vi "Big Temp Read and Test.vi"(7 "Initialize":bool, 8 "Error In":errorcluster, 9 "Cluster":T1, 10 "Cycle Time (S)":dbl, 11 "VISA resource name":refnum<visa-resource-name>) -> (0 "Error Out":errorcluster, 1 "Readout":dbl, 2 "Blinking":bool, 3 "VISA resource name":refnum<visa-resource-name>)   [LabVIEW 2021]
uses:
  <vilib>/Analysis/3filter.llb/Filter Passband Type.ctl
  <vilib>/Analysis/NI_AALBase.lvlib
  <vilib>/ptbypt/NI_PtbyPt.lvlib
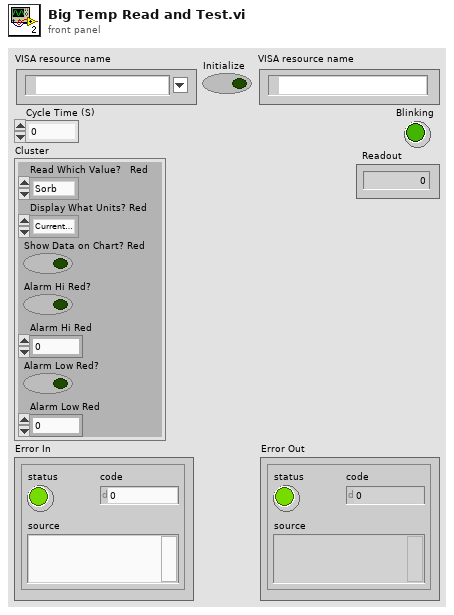
[diagram p1: front panel]
types:
  T1 = cluster{"Read Which Value?   Red":enum32{"Sorb", "1K Pot", "He3 Pot", "Probe"}, "Display What Units? Red":enum32{"Current Temperature", "Rate of Change"}, "Show Data on Chart? Red":bool, "Alarm Hi Red?":bool, "Alarm Hi Red":dbl, "Alarm Low Red?":bool, "Alarm Low Red":dbl}
  T2 = typedef "NI_AALBase.lvlib/Filter Passband Type.ctl" = enum32{"Lowpass", "Highpass", "Bandpass", "Bandstop"}
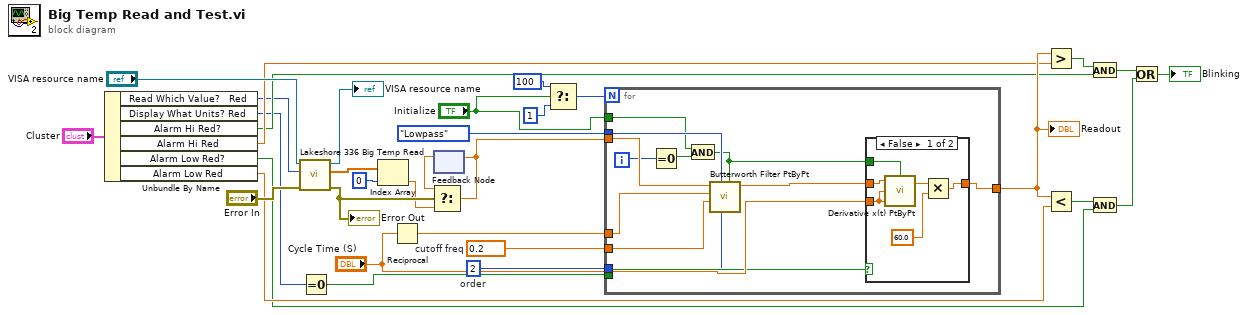
[diagram p0: block diagram]
diagram:
  w25 = 2  # order
  w28 = 0.2  # cutoff freq
  n1 = Unbundle By Name("Cluster") -> ("Read Which Value?   Red"=w6:enum32{"Sorb", "1K Pot", "He3 Pot", "Probe"}, "Display What Units? Red"=w13:enum32{"Current Temperature", "Rate of Change"}, "Alarm Hi Red?"=w14:bool, "Alarm Hi Red"=w15:dbl, "Alarm Low Red?"=w16:bool, "Alarm Low Red"=w17:dbl)
  n2 = call "Lakeshore 336 Big Temp Read.vi"("error in (no error)"="Error In", "Read Which Value?"=w6, "VISA Refnum in"="VISA resource name") -> ("error out"=w24:errorcluster, "Measurement"=w19:dbl[], "VISA Refnum out"=→"VISA resource name":refnum<visa-resource-name>)  [unwired: 6 in]
  "Error Out" <- w24
  n3 = Equal To 0?(x=w13) -> (x = 0?=w27:bool)
  n4 = Index Array(array=w19, index=0) -> (element=w5:dbl)
  n5 = Reciprocal(x="Cycle Time (S)") -> (1/x=w31:dbl)
  n6 = feedback #1() -> (w23:dbl)  [unwired: 1 in]
  n7 = Select(t=w23, s=w24, f=w5) -> (s? t:f=w26:dbl)
  n8 = feedback-in #1(w26) -> ()
  n9 = Select(t=100, s="Initialize", f=1) -> (s? t:f=w4:i32)
  n10 = for {
    N: w4 -> [_]
    tunnel: "Cycle Time (S)" -> [w45]
    tunnel: w31 -> [w44]
    tunnel: [w43] -> w30
    tunnel: Filter_Passband_Type."Lowpass" ("filter type") -> [w42]
    tunnel: "Initialize" -> [w34]
    tunnel: w28 -> [w41]
    tunnel: w27 -> [w40]
    tunnel: w26 -> [w38]
    tunnel: w25 -> [w37]
    i -> [w36]
    n11 = Equal To 0?(x=w36) -> (x = 0?=w35:bool)
    n12 = And(x=w34, y=w35) -> (x .and. y?=w33:bool)
    n13 = call <vilib>:"Butterworth Filter PtByPt.vi"("initialize"=w33, "order"=w37, "filter type"=w42, "high cutoff freq: fh"=w41, "sampling freq: fs"=w44, "x"=w38) -> ("Filtered x"=w39:dbl)  [unwired: 3 in, 1 out]
    n14 = case shown="False" w40 {
      tunnel: [w49 w52] -> w43
      tunnel: w39 -> [w51 w52]
      tunnel: w33 -> [w50 _]
      tunnel: w45 -> [w46 _]
      frame False {
        n15 = call <vilib>:"Derivative x(t) PtByPt.vi"("initialize"=w50, "dt"=w46, "initial condition"=w46, "x"=w51) -> ("dx/dt"=w48:dbl)  [unwired: 1 out]
        n16 = Multiply(x=w48, y=60.0) -> (x*y=w49:dbl)
      }
      frame True {
      }
    }
  }
  "Readout" <- w30
  n17 = Greater?(x=w30, y=w15) -> (0:w8:bool)
  n18 = Less?(x=w30, y=w17) -> (x < y?=w7:bool)
  n19 = And(x=w8, y=w14) -> (x .and. y?=w9:bool)
  n20 = And(x=w7, y=w16) -> (x .and. y?=w10:bool)
  n21 = Or(x=w9, y=w10) -> (x .or. y?=→"Blinking":bool)
